vi "3_Analog_Meter_Reader(Inference)_(Input_From_Control).vi"() -> ()   [LabVIEW 2020]
uses:
  Controls/Analog_Meter.ctl
  <vilib>/Ngene/Deep Learning Toolkit/Toolkit/NN_Network/Controls/NN_Save_Before_Destroy_Options.ctl
  <vilib>/Ngene/Deep Learning Toolkit/Toolkit/NN_Network/Controls/NN_Device.ctl
  <vilib>/Ngene/Deep Learning Toolkit/Toolkit/NN_Network/API/NN_Set_Input/3D/NN_Set_Input(3D_SGL_idx).vi
  <vilib>/Ngene/Deep Learning Toolkit/Toolkit/Deep_Learning_Toolkit_by_Ngene.lvlib
  <vilib>/vision/NI_Vision_Development_Module.lvlib
  <vilib>/ptbypt/NI_PtbyPt.lvlib
panel:
  out "Value":sgl=63.065025 format="%#.2g"
  out "Inference Time (ms)":dbl=0.002936366997892037 format="%#_3p"
  out "Ground Truth vs Prediction":cluster{sgl, "Numeric Control":sgl}(graph)
  out "Abs Error":sgl=0.1229247 format="%#_3g"
  out "Relative Error(%)":sgl=0.19529806 format="%#_3g"
  in  "Input":T1=62.94210062972307 scale=0.0..140.0
  out "Prediction":T1=63.065025329589844 scale=0.0..140.0
  out "Inference Speed (FPS)":dbl=340.55688567467257 format="%#_3p"
  in  "Stop":bool
  in  "Network Configuration File Path":path=path "D:/Ngene/GitHub/deepltk_examples/3_Image_Processing/31_Image_Regression/working/Analog_Meter/Analog_Meter_net_cfg_24_01_29__19_35_37.cfg"
  in  "Weight File Path":path=path "D:/Ngene/GitHub/deepltk_examples/3_Image_Processing/31_Image_Regression/working/Analog_Meter/Analog_Meter_weights_24_01_29__19_35_37.bin"
  # "Instructions:\n1. Provide model files (.cfg and .bin).\n2. Run the VI\n3. Manually move the arrow of Input Gauge and observe the presidcted Value."
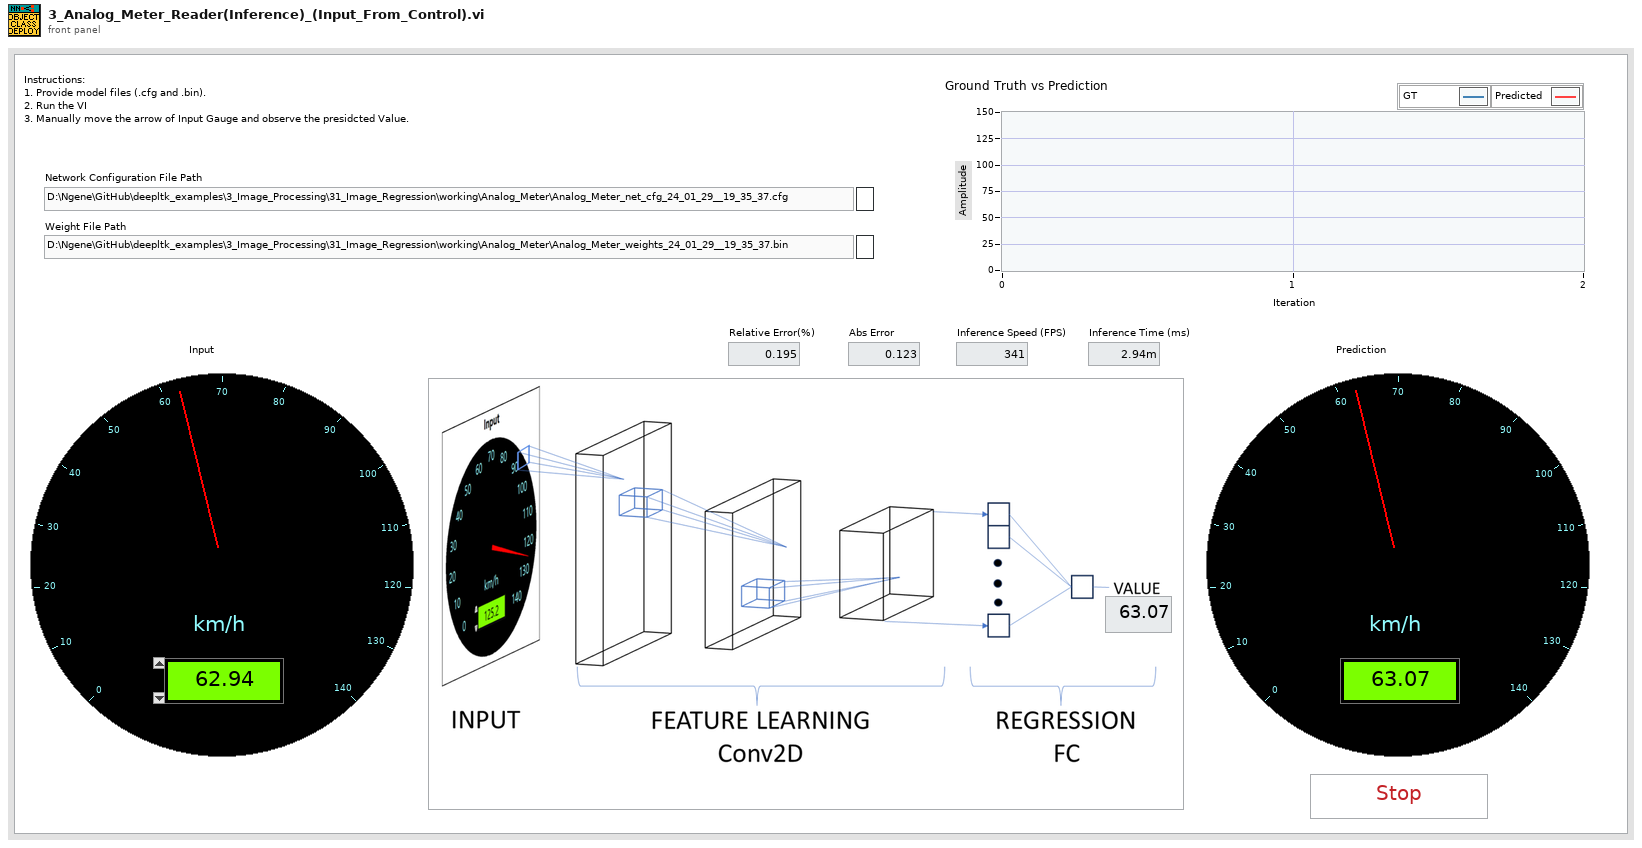
[diagram p1: front panel]
types:
  T1 = typedef "Analog_Meter.ctl" = dbl
  T2 = typedef "Image Type" = u32
  T3 = typedef "Deep_Learning_Toolkit_by_Ngene.lvlib/NN_Device.ctl" = enum16{"CPU", "GPU"}
  T4 = typedef "Deep_Learning_Toolkit_by_Ngene.lvlib/NN_Save_Before_Destroy_Options.ctl" = cluster{"CFG?":bool, "Weights?":bool, "Render?":bool}
  T5 = typedef "Deep_Learning_Toolkit_by_Ngene.lvlib/NN_Config_Params.ctl" = cluster{"Name":string, "mBatch":i32, "NN_Train_Params":T6, "LR_Decay_Policy":T9, "Labels":string[], "Loss":T11, "Max_WS_Size(B)":i64, "DryRun?":bool}
  T6 = typedef "Deep_Learning_Toolkit_by_Ngene.lvlib/NN_Train_Params.ctl" = cluster{"Optimizer":T7, "Beta_1":sgl, "Beta_2":sgl, "Weight Decay(L1)":sgl, "Weight Decay(L2)":sgl, "Data_Sampling":T8}
  T7 = typedef "Deep_Learning_Toolkit_by_Ngene.lvlib/NN_Train_Optimizer.ctl" = enum16{"SGD", "Adam", "Adagrad", "Adadelta", "RMSProp", "Nesterov"}
  T8 = typedef "Deep_Learning_Toolkit_by_Ngene.lvlib/NN_Train_Data_Sampling.ctl" = enum16{"Random", "Sequential"}
  T9 = typedef "Deep_Learning_Toolkit_by_Ngene.lvlib/NN_LR_Policy_Cfg.ctl" = cluster{"Policy_Type":T10, "LR0":dbl, "k":sgl, "WarmUp_Policy":enum16{"Step", "Ramp"}, "WarmUp_Iter":i32, "WarmUp_Ratio":sgl}
  T10 = typedef "Deep_Learning_Toolkit_by_Ngene.lvlib/NN_LR_Policy_Type.ctl" = enum16{"Manual", "Step", "Exp", "1/t"}
  T11 = typedef "Deep_Learning_Toolkit_by_Ngene.lvlib/NN_Loss_Config_Params.ctl" = cluster{"Loss_Type":T12, "Loss_Conf_Params":variant}
  T12 = typedef "Deep_Learning_Toolkit_by_Ngene.lvlib/NN_Loss_Type.ctl" = enum16{"None", "MSE", "CrossEntropy", "YOLO_v2", "YOLO_v4"}
  T13 = typedef "Deep_Learning_Toolkit_by_Ngene.lvlib/NN_Layer_Config_Params.ctl" = cluster{"Layer_Type":T14, "Layer_Conf_Params":variant, "Input Layers":string[]}
  T14 = typedef "Deep_Learning_Toolkit_by_Ngene.lvlib/NN_Layer_Type.ctl" = enum16{"Input1D", "Input3D", "Conv1D", "Conv2D", "Conv2D_Adv", "MaxPool", "AvgPool", "UpSample", "DropOut3D", "ShortCut", "Concat", "SoftMax3D", "FC", "DropOut", "Softmax", "Flatten", "YOLO_v2", "YOLO_v4", "Activation", "BatchNormalization", "LayerNormalization", "Scale", "Unsupported"}
  T15 = typedef "Deep_Learning_Toolkit_by_Ngene.lvlib/NN.ctl" = cluster{"Name":string, "No of Layers":i32, "mBatch":i32, "Layers":T16[], "Dimty":T17, "Dims_In":T18, "Dims_Out":T18, "Working_Dir":path, "Train?":bool, "Train_Params":T6, "LR_Update_Policy":T9, "Session Data":T19, "Ground_truth":T20, "NNg_hdls":T21, "NN_Device":T3, "GPU Id":i32, "Labels":string[], "Loss_Type":T12, "Loss_Cfg_Prms":variant, "NNG_WS":T22, "DryRun?":bool}
  T16 = typedef "Deep_Learning_Toolkit_by_Ngene.lvlib/NN_Layer_ref.ctl" = refnum<file>
  T17 = typedef "Deep_Learning_Toolkit_by_Ngene.lvlib/NN_In_Out_Dim-ty.ctl" = enum8{"In1D_Out1D", "In3D_Out1D", "In3D_Out3D", "In3D_OutBBox"}
  T18 = typedef "Deep_Learning_Toolkit_by_Ngene.lvlib/NN_Dims(C,H,W).ctl" = cluster{"C":i32, "H":i32, "W":i32}
  T19 = typedef "Deep_Learning_Toolkit_by_Ngene.lvlib/NN_Train_Session_Data.ctl" = cluster{"Epochs":sgl, "Tot_Iter":i32, "LR":sgl, "LR_iter":i32}
  T20 = typedef "Deep_Learning_Toolkit_by_Ngene.lvlib/NN_Ground_truth.ctl" = cluster{"Y":variant}
  T21 = typedef "Deep_Learning_Toolkit_by_Ngene.lvlib/nng_cuda_handles.ctl" = cluster{"cudnn":u64, "cublas":u64, "stream":u64, "curand":u64}
  T22 = typedef "Deep_Learning_Toolkit_by_Ngene.lvlib/NNG_WS.ctl" = cluster{"NNG_WS_Mem":T23, "Max_WS_Size":i64}
  T23 = typedef "Deep_Learning_Toolkit_by_Ngene.lvlib/NNg_WS_Mem_DVR.ctl" = refnum<data-value>
  T24 = typedef "IMAQ Image.ctl" = refnum<image>
  T25 = typedef "imagedata.ctl" = cluster{"image type":i32, "image depth":i32, "image":u8[], "mask":u8[], "colors":u32[], "Rectangle":cluster{"left":i16, "top":i16, "right":i16, "bottom":i16}}
  T26 = typedef "Deep_Learning_Toolkit_by_Ngene.lvlib/NN_Layer.ctl" = cluster{"Name":string, "Layer_Data":T27, "Layer_Type":T14, "Dims_In":T18, "Layers_In":T16[], "Dims_Out":T18, "Layers_Out":T16[], "Metrics":T28, "GPU_Data":T29, "mBatch":i32, "NN_Device":T3, "NNg_hdls":T21, "Train?":bool, "Dimty":T30, "RecptField":T31, "Idx":i32}
  T27 = typedef "Deep_Learning_Toolkit_by_Ngene.lvlib/NN_Layer_Data_Refnum.ctl" = refnum<file>
  T28 = typedef "Deep_Learning_Toolkit_by_Ngene.lvlib/NN_Layer_Metrics.ctl" = cluster{"Data":dbl, "Params":dbl, "Ops":dbl}
  T29 = typedef "Deep_Learning_Toolkit_by_Ngene.lvlib/NNg_Layer_Data_Refnum.ctl" = refnum<file>
  T30 = typedef "Deep_Learning_Toolkit_by_Ngene.lvlib/NN_Layer_Dimty.ctl" = enum16{"1D", "3D"}
  T31 = typedef "Deep_Learning_Toolkit_by_Ngene.lvlib/NN_Layer_RF_State.ctl" = cluster{"Dims":T32, "J":T32}
  T32 = typedef "Deep_Learning_Toolkit_by_Ngene.lvlib/NN_Dims(V,H).ctl" = cluster{"V":i32, "H":i32}
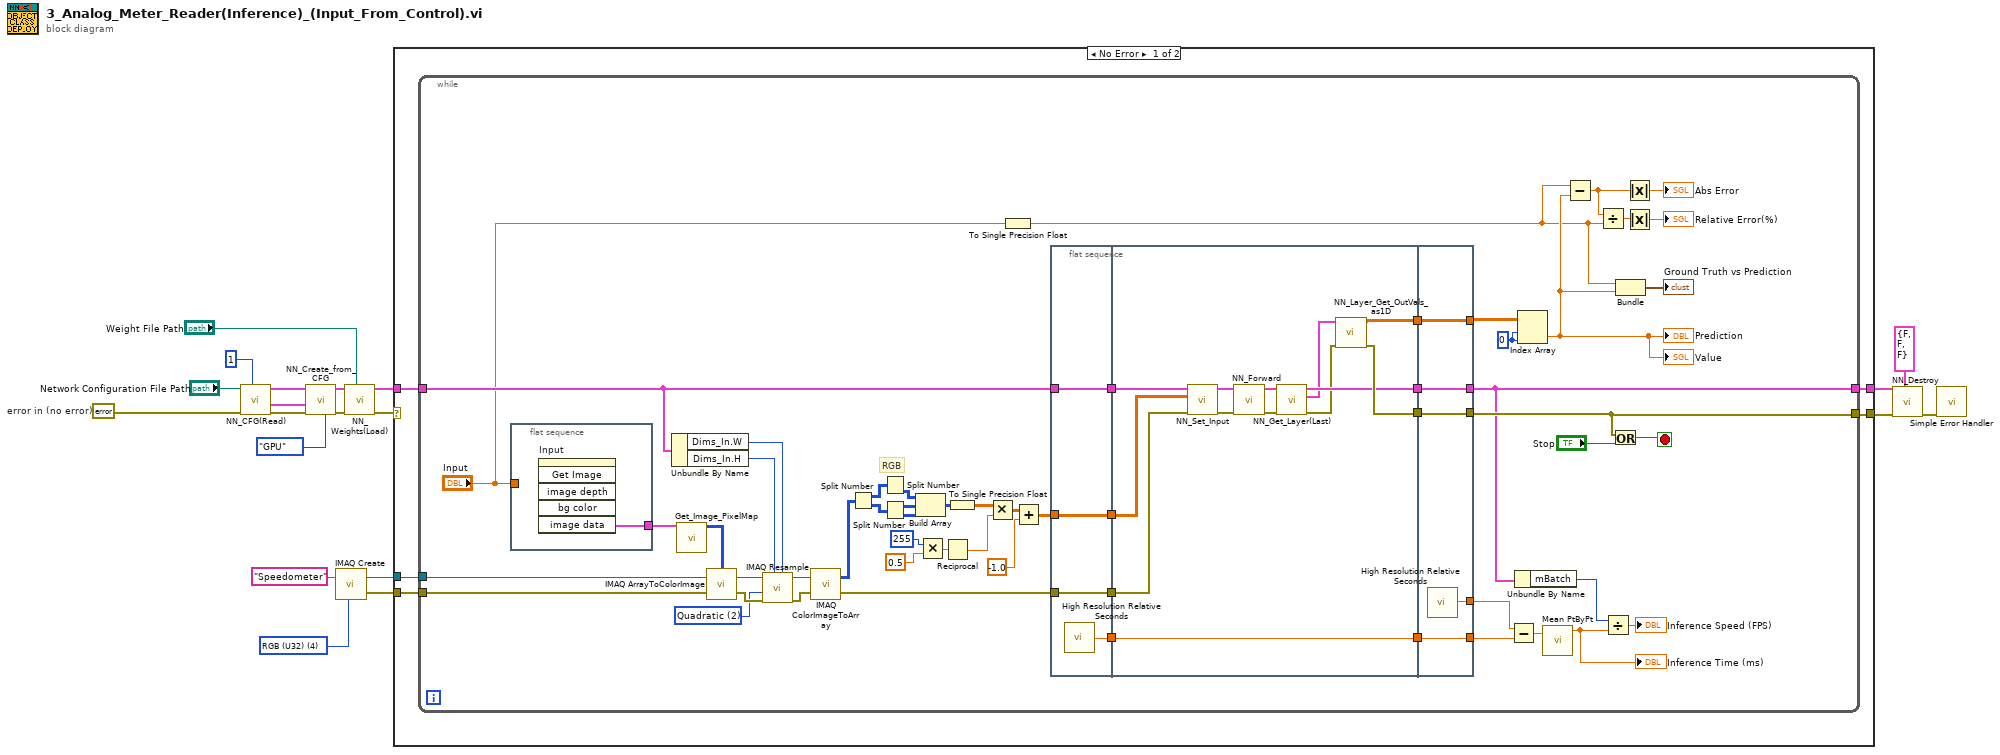
[diagram p0: block diagram]
diagram:
  w2 = T2 4 items=["Grayscale (U8)", "Grayscale (I16)", "Grayscale (SGL)", "Complex (CSG)", "RGB (U32)", "HSL (U32)", "RGB (U64)", "Grayscale (U16)"] ("Image Type")
  w10 = errorcluster {"status"=FALSE, "code"=0, "source"=""}  # error in (no error)
  n1 = call <vilib>:"NN_CFG(Read).vi"("mBatch"=1, "error in (no error)"=w10, "CFG file path"="Network Configuration File Path") -> ("error out"=w20:errorcluster, "Net_Cfg"=w8:T5, "Layer_Cfg"=w13:T13[])  [unwired: 6 in]
  n2 = call <vilib>:"NN_Create_from_CFG.vi"("NN_Device"=NN_Device."GPU", "error in (no error)"=w20, "Net_Cfg"=w8, "Layer_Cfg"=w13) -> ("error out"=w15:errorcluster, "NN out"=w12:T15)  [unwired: 6 in]
  n3 = call "IMAQ Create"("Image Name"="Speedometer", "Image Type"=w2) -> ("New Image"=w4:T24, "error out"=w3:errorcluster)  [unwired: 3 in]
  n4 = call <vilib>:"NN_Weights(Load).vi"("Weight File Path"="Weight File Path", "error in (no error)"=w15, "NN in"=w12) -> ("error out"=w9:errorcluster, "NN out"=w11:T15)  [unwired: 7 in]
  n5 = case shown="No Error" w9 {
    selector: w9 -> [_ w105]
    tunnel: w11 -> [w25 w106]
    tunnel: [w24 w106] -> w18
    tunnel: [w23 w105] -> w17
    tunnel: w4 -> [w22 _]
    tunnel: w3 -> [w21 _]
    frame No Error {
      n6 = while {
        tunnel: w25 -> [w56]
        tunnel: [w78] -> w24
        tunnel: [w79] -> w23
        tunnel: w22 -> [w53]
        tunnel: w21 -> [w52]
        stop <- w80 stop-if-true
        w60 = 0 ("disabled index (col)")
        w63 = u32 2 items=["Zero Order", "Bi-Linear", "Quadratic", "Cubic Spline"] ("Interpolation Type")
        # "RGB"
        n7 = flat-sequence {
          tunnel: [w82] -> w65
          tunnel: "Input" -> [_]
          frame #0 {
            n8 = invoke on="Input" class="Knob (strict)" method="Get Image"() -> ("image data"=w82:T25)  [unwired: 6 in, 5 out]
          }
        }
        n9 = Unbundle By Name(w56) -> ("Dims_In.W"=w54:i32, "Dims_In.H"=w55:i32)
        n10 = call "Get_Image_PixelMap.vi"("Image Data"=w65) -> ("Image PixelMap"=w67:u32[][])  [unwired: 10 in]
        n11 = call "IMAQ ArrayToColorImage"("Image Pixels (U32)"=w67, "Image"=w53, "error in (no error)"=w52) -> ("Image Out"=w64:T24, "error out"=w66:errorcluster)  [unwired: 2 in]
        n12 = call "IMAQ Resample"("X Resolution"=w54, "Y Resolution"=w55, "error in (no error)"=w66, "Interpolation Type"=w63, "Image Src"=w64) -> ("error out"=w62:errorcluster, "Image Dst Out"=w61:T24)  [unwired: 5 in]
        n13 = call "IMAQ ColorImageToArray"("Image"=w61, "error in (no error)"=w62) -> ("Image Pixels (U32)"=w51:u32[][], "error out"=w76:errorcluster)  [unwired: 2 in, 1 out]
        n14 = Split Number(x=w51) -> (hi(x)=w49:u16[][], lo(x)=w50:u16[][])
        n15 = Split Number(x=w49) -> (lo(x)=w47:u8[][])  [unwired: 1 out]
        n16 = Split Number(x=w50) -> (hi(x)=w46:u8[][], lo(x)=w45:u8[][])
        n17 = Build Array(w47, w46, w45) -> (w48:u8[][][])
        n18 = Multiply(x=u16 255 ("dimension size"), y=sgl 0.5 ("dimension size")) -> (x*y=w43:sgl)
        n19 = Reciprocal(x=w43) -> (1/x=w44:sgl)
        n20 = To Single Precision Float(number=w48) -> (single precision float=w38:sgl[][][])
        n21 = Multiply(x=w38, y=w44) -> (x*y=w42:sgl[][][])
        n22 = To Single Precision Float(number="Input") -> (single precision float=w26:sgl)
        n23 = Add(x=w42, y=sgl -1.0 ("dimension size")) -> (x+y=w36:sgl[][][])
        n24 = flat-sequence {
          tunnel: w76 -> [w85]
          tunnel: w56 -> [w86]
          tunnel: [w86] -> w75
          tunnel: [w85] -> w74
          tunnel: [w84] -> w37
          tunnel: w36 -> [w84]
          tunnel: [w83] -> w33
          tunnel: w75 -> [w98]
          tunnel: w74 -> [w89]
          tunnel: [w99] -> w73
          tunnel: [w97] -> w72
          tunnel: [w96] -> w71
          tunnel: w37 -> [w88]
          tunnel: [w87] -> w34
          tunnel: w33 -> [w87]
          tunnel: [w102] -> w78
          tunnel: [w103] -> w79
          tunnel: [w104] -> w81
          tunnel: w73 -> [w104]
          tunnel: w72 -> [w103]
          tunnel: w71 -> [w102]
          tunnel: [w101] -> w70
          tunnel: [w100] -> w35
          tunnel: w34 -> [w100]
          frame #0 {
            n25 = call <vilib>:"High Resolution Relative Seconds.vi"() -> ("relative seconds"=w83:dbl)
          }
          frame #1 {
            n26 = call-poly <vilib>:"NN_Set_Input.vi"("error in (no error)"=w89, "Data_In(3D_SGL)"=w88, "NN in"=w98) -> ("error out"=w93:errorcluster, "NN out"=w92:T15)  [unwired: 7 in]
            n27 = call <vilib>:"NN_Forward.vi"("error in (no error)"=w93, "NN in"=w92) -> ("error out"=w91:errorcluster, "NN out"=w90:T15)  [unwired: 6 in, 2 out]
            n28 = call <vilib>:"NN_Get_Layer(Last).vi"("error in (no error)"=w91, "NN in"=w90) -> ("error out"=w95:errorcluster, "Last_Layer"=w94:T26, "NN out"=w96:T15)  [unwired: 6 in, 1 out]
            n29 = call <vilib>:"NN_Layer_Get_OutVals_as1D.vi"("error in (no error)"=w95, "Layer"=w94) -> ("error out"=w97:errorcluster, "Out(as1D)"=w99:sgl[][])  [unwired: 8 in]
          }
          frame #2 {
            n30 = call <vilib>:"High Resolution Relative Seconds.vi"() -> ("relative seconds"=w101:dbl)
          }
        }
        n31 = Subtract(x=w70, y=w35) -> (x-y=w30:dbl)
        n32 = Unbundle By Name(w78) -> ("mBatch"=w77:i32)
        n33 = Index Array(array=w81, index (row)=w60, index (col)=w60) -> (element=w28:sgl)
        "Prediction" <- w28
        "Value" <- w28
        n34 = call <vilib>:"Mean PtByPt.vi"("x"=w30) -> ("mean"=w29:dbl)  [unwired: 3 in, 1 out]
        "Inference Time (ms)" <- w29
        n35 = Subtract(x=w26, y=w28) -> (x-y=w58:sgl)
        n36 = Divide(x=w58, y=w26) -> (x/y=w59:sgl)
        n37 = Divide(x=w77, y=w29) -> (x/y=→"Inference Speed (FPS)":dbl)
        n38 = Or(x=w79, y="Stop") -> (x .or. y?=w80:bool)
        n39 = Bundle(w26, "Numeric Control"=w28) -> (→"Ground Truth vs Prediction":cluster{sgl, "Numeric Control":sgl})  [unwired: 1 in]
        n40 = Absolute Value(x=w58) -> (abs(x)=→"Abs Error":sgl)
        n41 = Absolute Value(x=w59) -> (abs(x)=→"Relative Error(%)":sgl)
      }
    }
    frame Error {
    }
  }
  n42 = call <vilib>:"NN_Destroy.vi"("Save (T, T, T)"=T4 {"CFG?"=FALSE, "Weights?"=FALSE, "Render?"=FALSE} ("Save_Config"), "error in (no error)"=w17, "NN in"=w18) -> ("error out"=w1:errorcluster)  [unwired: 7 in, 1 out]
  n43 = call <vilib>:"Simple Error Handler.vi"("error in (no error)"=w1) -> ()  [unwired: 4 in, 5 out]
